vi "DataWriterFactory.vi"() -> ()   [LabVIEW 2024, in "Data.lvlib"]
uses:
  Data.lvlib
  Data/DataModel/MeasurementData.ctl
  Controls/SensorType.ctl
  Controls/Config.ctl
  TXT_Writer/TXT_Writer.lvclass
  TXT_Writer/TXT_Writer.lvclass/TXT_Writer.ctl
  Sensors.lvlib
panel:
  out "error out":errorcluster
  in  "MeasurementData":T1
  in  "Path":path
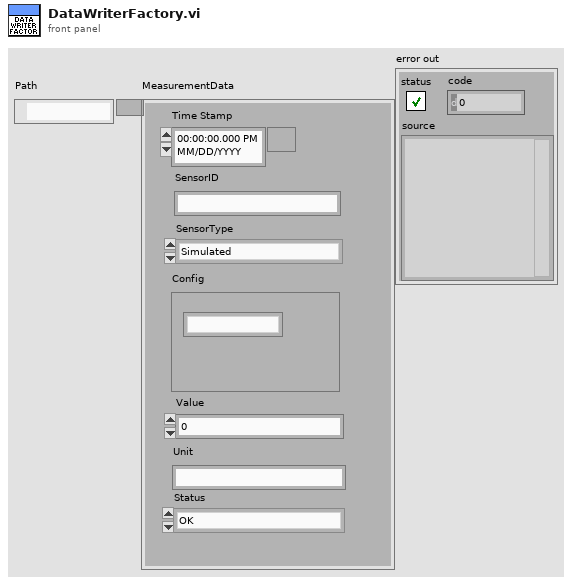
[diagram p1: front panel]
types:
  T1 = typedef "Data.lvlib/MeasurementData.ctl" = cluster{"Time Stamp":timestamp, "SensorID":string, "SensorType":T2, "Config":T3, "Value":dbl, "Unit":string, "Status":enum16{"OK", "Warning", "Error"}}
  T2 = typedef "Sensors.lvlib/SensorType.ctl" = enum16{"Simulated", "pH", "NPK"}
  T3 = typedef "Sensors.lvlib/Config.ctl" = cluster{"String":string}
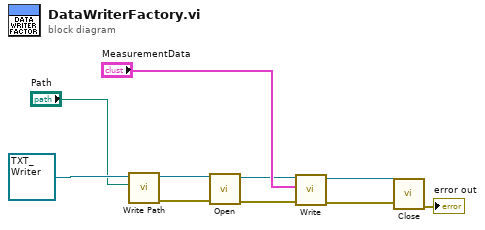
[diagram p0: block diagram]
diagram:
  n1 = call "Write Path.vi"("Path"="Path", "TXT_Writer in"=refnum<class "TXT_Writer.lvclass"> refnum) -> ("error out"=w3:errorcluster, "TXT_Writer out"=w4:refnum<class "TXT_Writer.lvclass">)  [unwired: 8 in]
  n2 = call-dynamic "Open.vi"("error in (no error)"=w3, "TXT_Writer in"=w4) -> ("error out"=w2:errorcluster, "TXT_Writer out"=w1:refnum<class "TXT_Writer.lvclass">)  [unwired: 8 in]
  n3 = call-dynamic "Write.vi"("error in (no error)"=w2, "MeasurementData"="MeasurementData", "TXT_Writer in"=w1) -> ("error out"=w9:errorcluster, "TXT_Writer out"=w8:refnum<class "TXT_Writer.lvclass">)  [unwired: 7 in]
  n4 = call-dynamic "Close.vi"("error in (no error)"=w9, "TXT_Writer in"=w8) -> ("error out"=→"error out":errorcluster)  [unwired: 8 in, 1 out]
